vi "3_AdvancedDemo_HHT3.vi"() -> ()   [LabVIEW 2010]
uses:
  Types/HH_UIThread_Data.ctl
  Types/HH_InputChannel.ctl
  _lib/PQ/HydraHarp/HH_RefSource.ctl
  _lib/PQ/HydraHarp/HH_MeasMode.ctl
  _lib/PQ/HydraHarp/hhlib_x86_x64_UIThread.llb/HH_DllPath_global.vi
  <vilib>/Utility/error.llb/DialogType.ctl
  Types/HH_DataProcThread_QCmds.ctl
  Types/HH_DataProcThread_QData.ctl
  Types/HH_VisThread_QCmds.ctl
  Types/HH_VisThread_QData.ctl
  Types/HH_VisThread_Data.ctl
  _lib/PQ/HydraHarp/HH_LibVersion_global.vi
  _lib/PQ/HydraHarp/HH_InitInfo.ctl
  Types/HH_UIThread_Cmds.ctl
panel:
  in  "Settings":bool=TRUE
  in  "Run continuously":bool caption="Conti."
  in  "Start":bool
  in  "Scale":bool
  out "CountRates":i32[](graph)
  in  "HistoAcqTime":dbl=1.0 caption="Int.Time    s" min=0.1 max=360000.0 step=0.1
  in  "AcqTime":i32=360000000 caption="T3Acq.   ms" min=1 max=360000 step=1
  in  "Binning":i32(ring) caption="Resol.      ps" items=["1", "2", "4", "8", "16", "32", "64", "128", "256", "512", "1024", "2048", "4096", "8192", "16384", "32768", "65536", "131072", "262144", "524288", "1048576", "2097152", "4194304", "8388608", "16777216", "33554432"]
  in  "HistoOffset":i32 caption="Offset      ns" min=0 max=500000 step=1
  out "DeltaT":dbl=inf caption="Resol.     ms" format="%.2f"
  in  "BitShift":i32=15 min=0 max=32 step=1
  in  "OvlLevel":i32=65536 caption="Ovl.Level" min=1024 max=65536 step=1024
  in  "StopOvl.":bool=TRUE
  out "TTraceGraph":T1(graph)
  out "HistoGraph":cluster{dbl, "Resol":dbl, "Histos":u32[][]}(graph)
  in  "SyncZeroX":i32=10 caption="ZeroCr.  mV" min=0 max=40 step=1
  in  "SyncDivider":i32(ring)=3 caption="Divider" items=["1", "2", "4", "8", "16"]
  in  "SyncOffset":i32 caption="Offset      ps" min=-99999 max=99999 step=1
  in  "SyncLevel":i32=50 caption="Level      mV" min=0 max=1000 step=1
  in  "Channels":T2[](array[typedef])=[{"Name"="Inp.Chan 1", "Enable"=TRUE, "Offset"=0, "CFDLevel"=50, "ZeroX"=10}, {"Name"="Inp.Chan 2", "Enable"=TRUE, "Offset"=0, "CFDLevel"=50, "ZeroX"=10}, {"Name"="Inp.Chan 3", "Enable"=TRUE, "Offset"=0, "CFDLevel"=50, "ZeroX"=10}, {"Name"="Inp.Chan 4", "Enable"=TRUE, "Offset"=0, "CFDLevel"=50, "ZeroX"=10}, {"Name"="Inp.Chan 5", "Enable"=TRUE, "Offset"=0, "CFDLevel"=50, "ZeroX"=10}, {"Name"="Inp.Chan 6", "Enable"=TRUE, "Offset"=0, "CFDLevel"=50, "ZeroX"=10}, {"Name"="Inp.Chan 7", "Enable"=TRUE, "Offset"=0, "CFDLevel"=50, "ZeroX"=10}, {"Name"="Inp.Chan 8", "Enable"=TRUE, "Offset"=0, "CFDLevel"=50, "ZeroX"=10}] {"ZeroX" min=0 max=40 step=1; "Offset" min=-99999 max=99999 step=1; "CFDLevel" min=0 max=1000 step=1}
  out "SyncRate":string="Sync Rate: 0 cps\n"
  out "OverRun":bool caption="Overrun:"
  out "Status":string="Elements in Q: 0"
  # "Histogram"
  # "Time Trace"
  # "Sync"
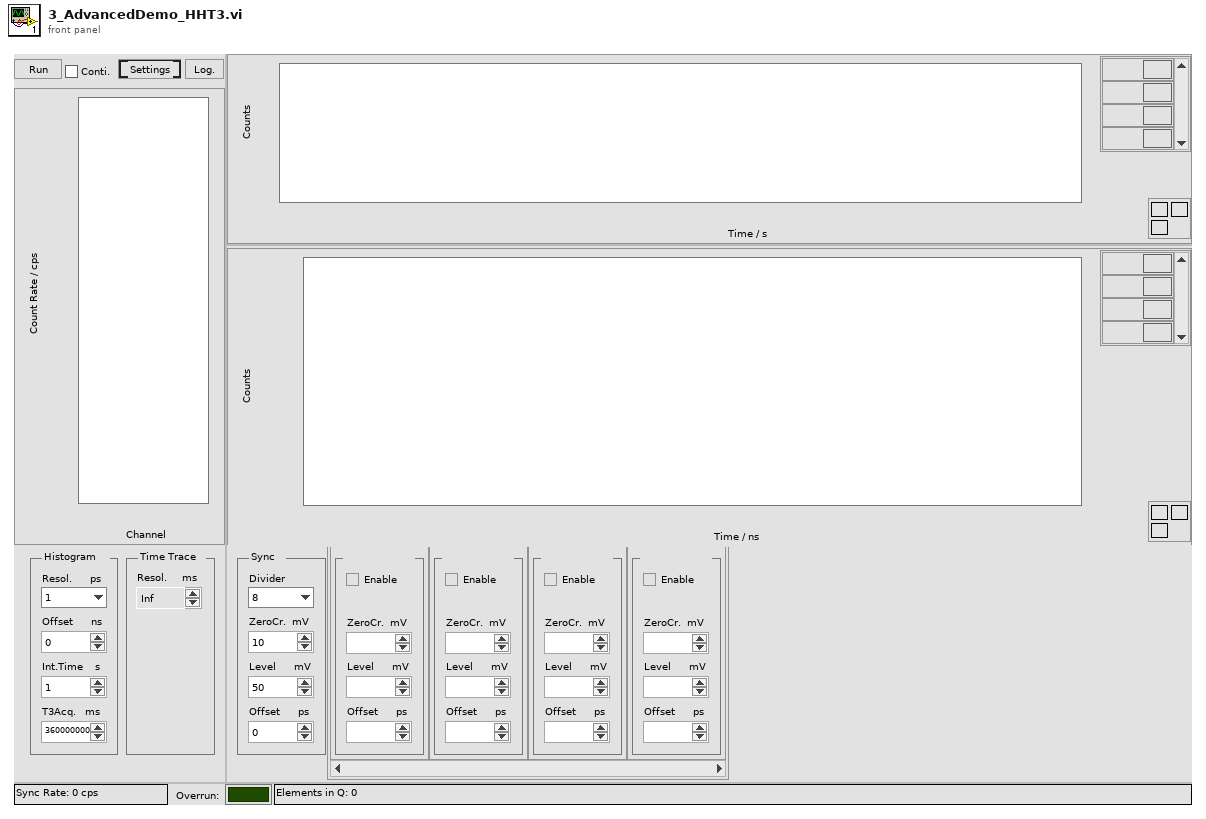
[diagram p1: front panel]
types:
  T1 = cluster{dbl, "Resolution":dbl, "Histogram":u32[][]}
  T2 = typedef "HH_InputChannel.ctl" = cluster{"Name":string, "Enable":bool, "Offset":i32, "CFDLevel":i32, "ZeroX":i32}
  T3 = typedef "HH_DataProcThread_QCmds.ctl" = enum16{"Exit", "Proc", "Init", "SetShift", "SetNumChannels", "SetHistAcqTime"}
  T4 = typedef "HH_VisThread_Data.ctl" = cluster{"Resol":dbl, "DeltaT":dbl, "NumChannels":i32}
  T5 = typedef "HH_VisThread_QData.ctl" = cluster{"Histos":u32[][], "Cmd":T6, "TimeTrace":u32[][], "Bin":i32, "Total bin":u64, "Status":string, "Resol":dbl, "DeltaT":dbl, "nChannels":i32}
  T6 = typedef "HH_VisThread_QCmds.ctl" = enum16{"_none_", "Resol", "nChannels", "DeltaT", "Histo", "TTrace", "Status"}
  T7 = typedef "HH_DataProcThread_QData.ctl" = cluster{"Cmd":T3, "nActual":i32, "Buffer":u32[], "TickCount":u32, "Param":i32}
  T8 = typedef "HH_UIThread_Data.ctl" = cluster{"Init Info":T9, "DevIdx":i32, "SyncDivider":i32, "SyncOffset":i32, "SyncLevel":i32, "Channels":T2[], "CurrentChannels":i32[], "AcqTime":i32, "Binning":i32, "HistoOffset":i32, "HistoLen":i32, "StopOvl.":bool, "OvlLevel":u32, "StartMeas":bool, "HistoLength":i32, "Resolution":dbl, "Run cont.":bool, "Status":string, "SyncRate":i32, "BitShift":i32, "HistoAcqTime":dbl, "SyncZeroX":i32, "SyncRateStart":i32}
  T9 = typedef "HH_InitInfo.ctl" = cluster{"Library Version":string, "Serial No.":string, "Model":string, "Partnum":string, "Version":string, "features":i32, "nchannels":i32, "nummod":i32, "Model Codes":i32[], "Version Codes":i32[], "Base Resolution":dbl, "Bin Steps":i32}
  T10 = typedef "HH_UIThread_Cmds.ctl" = enum16{"Idle", "Init", "SetInpChanEnable", "SetInpChanOffset", "SetInpChanTrg", "SetSyncDivider", "SetSyncTrg", "SetSyncOffset", "SetBinning", "SetHistoOffset", "SetHistoLen", "SetStopOvl", "SetBitShift", "SetHistoAcqTime", "GetRates", "StartMeas", "StopMeas", "AbortMeas", "GetResolution", "GetHisto", "ReadFiFo", "WriteStatus", "Resize", "EnableControls", "DisableControls", "Error", "Exit"}
  T11 = enum8{"Enabled", "Disabled", "Disabled and Grayed Out"}
  T12 = typedef "HH_MeasMode.ctl" = i32
  T13 = typedef "HH_RefSource.ctl" = enum16{"internal", "external"}
  T14 = typedef "DialogType.ctl" = u16
  T15 = cluster{"T0":dbl, "dt":dbl, "TimeTrace_out":u32[][]}
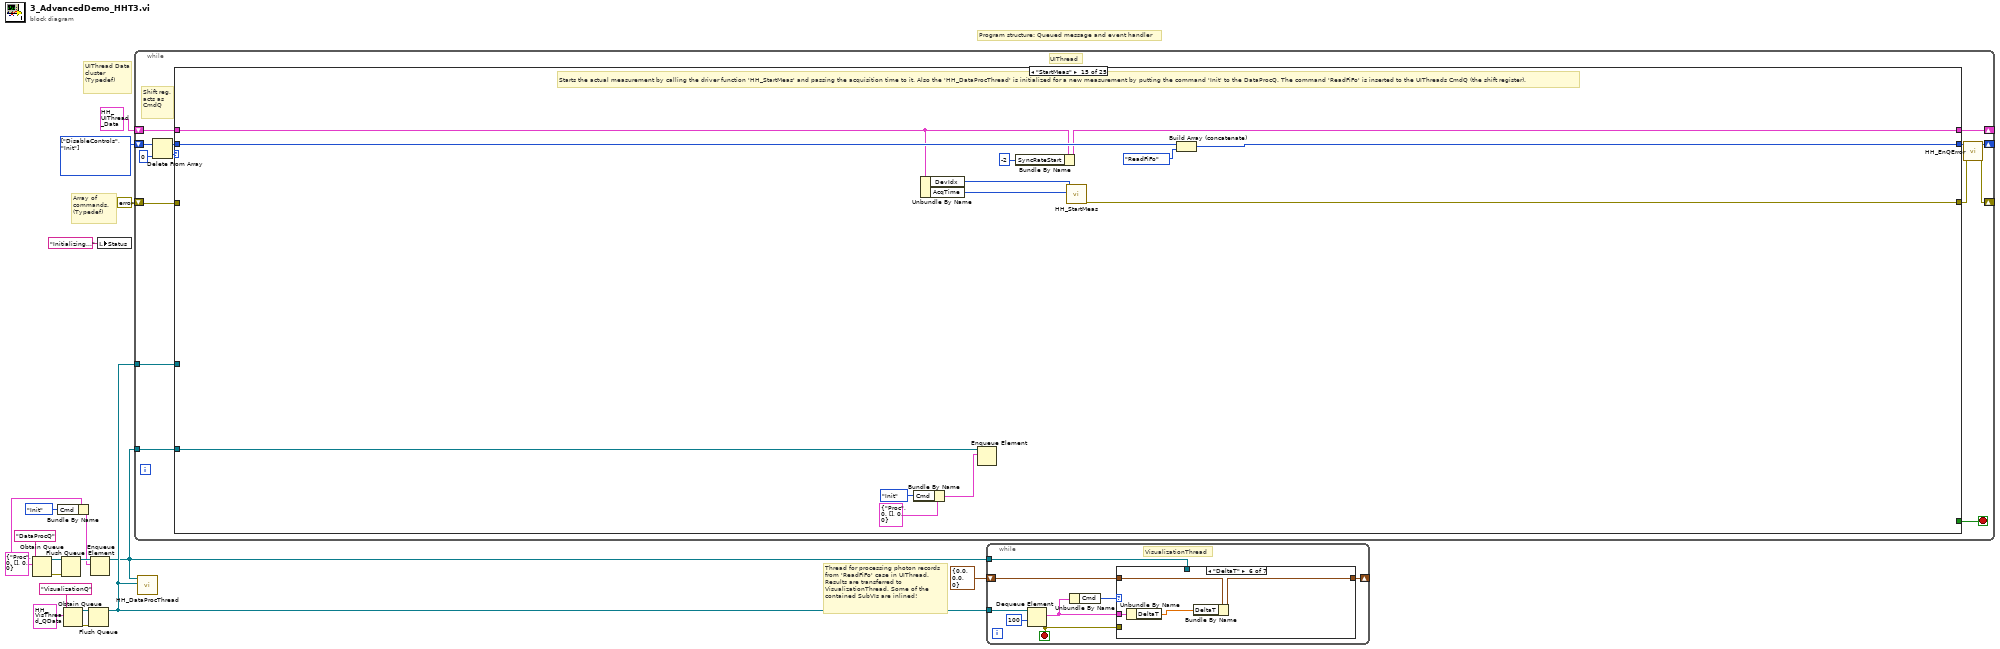
[diagram p0: block diagram]
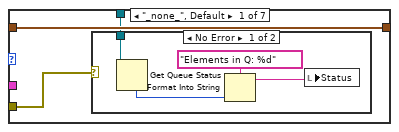
[diagram p2: hidden frame]
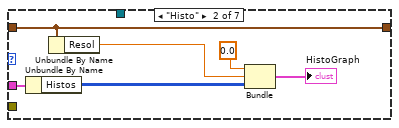
[diagram p4: hidden frame]
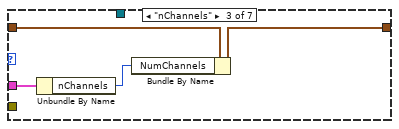
[diagram p5: hidden frame]
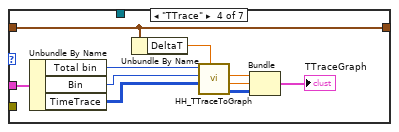
[diagram p6: hidden frame]
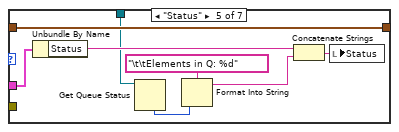
[diagram p7: hidden frame]
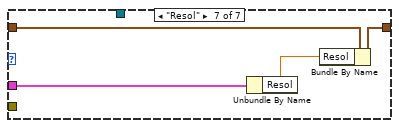
[diagram p8: hidden frame]
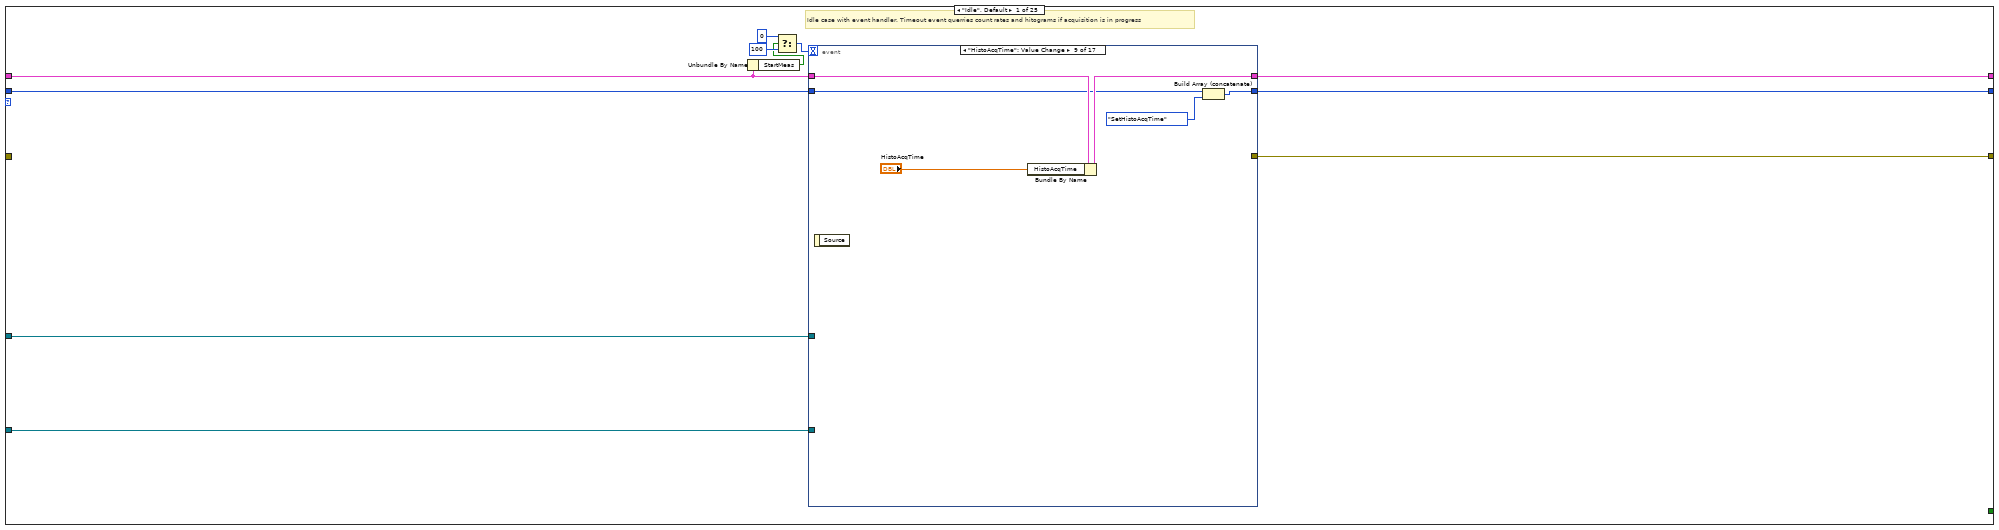
[diagram p9: hidden frame]
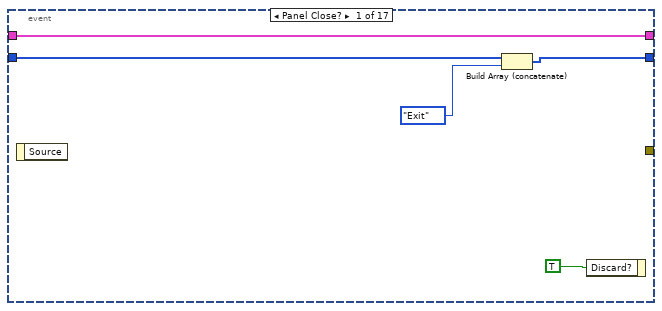
[diagram p10: hidden frame]
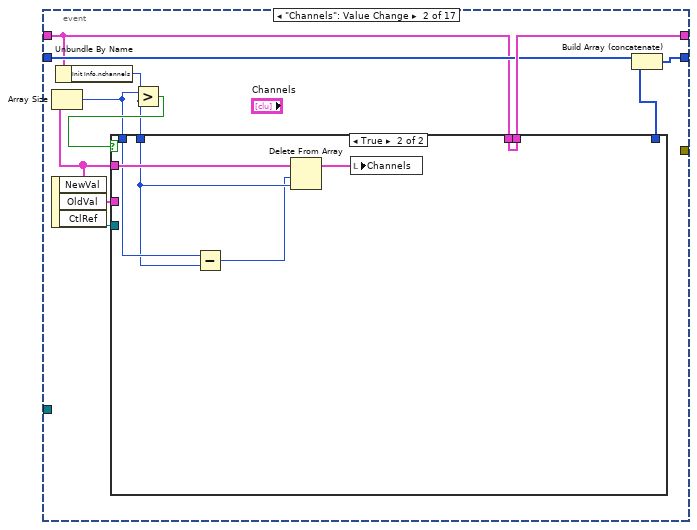
[diagram p11: hidden frame]
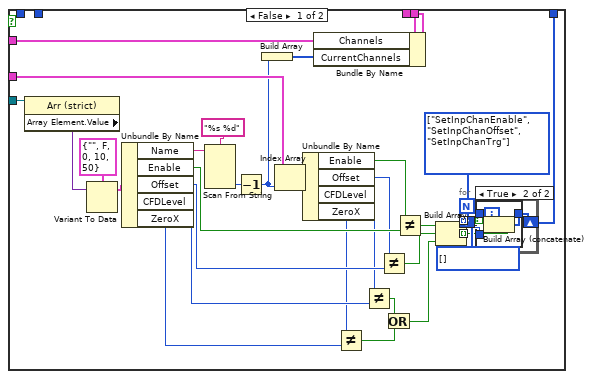
[diagram p12: hidden frame]
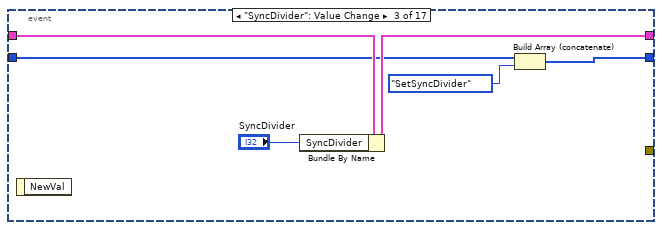
[diagram p14: hidden frame]
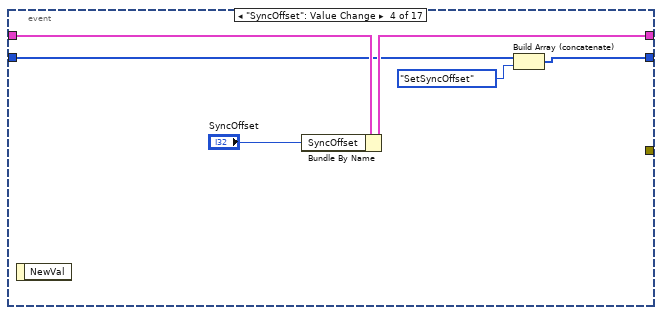
[diagram p15: hidden frame]
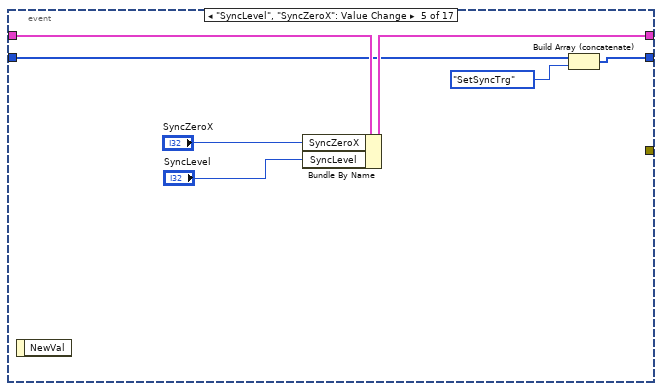
[diagram p16: hidden frame]
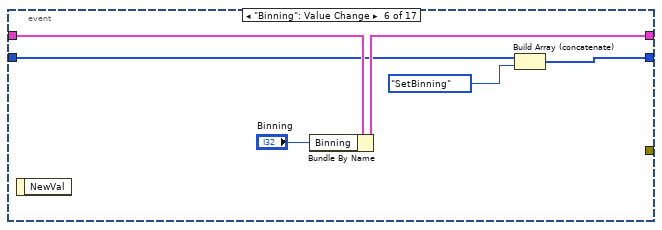
[diagram p17: hidden frame]
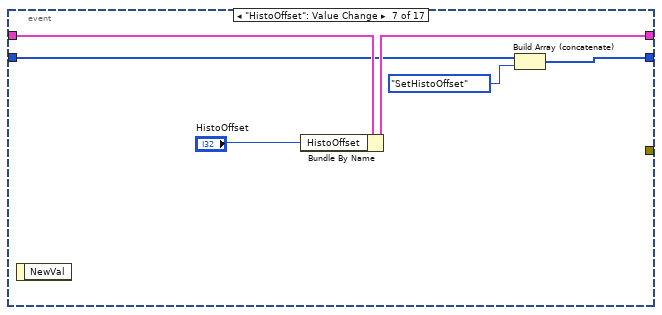
[diagram p18: hidden frame]
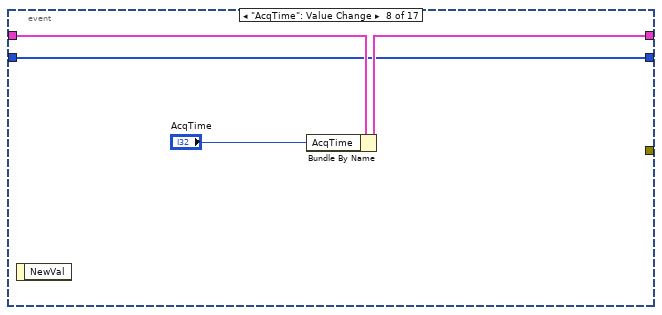
[diagram p19: hidden frame]
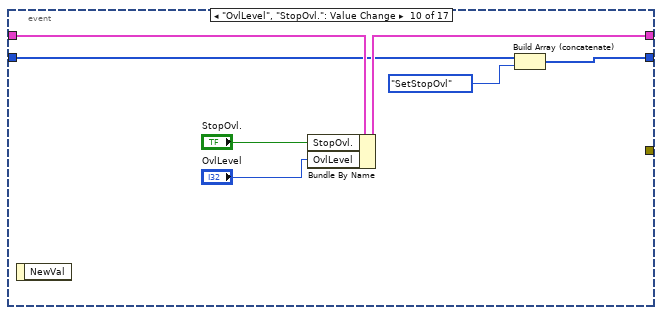
[diagram p20: hidden frame]
diagram:
  w4 = T7 {"Cmd"=enum."Proc", "nActual"=0, "Buffer"=[], "TickCount"=0, "Param"=0} ("MH_DataProcThread_QData")
  w17 = T10[] [enum."DisableControls", enum."Init"] items=["Idle", "Init", "SetInpChanEnable", "SetInpChanOffset", "SetInpChanTrg", "SetSyncDivider", "SetSyncTrg", "SetSyncOffset", "SetBinning", "SetHistoOffset", "SetHistoLen", "SetStopOvl", "SetBitShift", "SetHistoAcqTime", "GetRates", "StartMeas", "StopMeas", "AbortMeas", "GetResolution", "GetHisto", "ReadFiFo", "WriteStatus", "Resize", "EnableControls", "DisableControls", "Error", "Exit"]
  # "Thread for processing photon records from 'ReadFiFo' case in UIThread. Results are transferred to VisualizationThread. Some of the contained SubVIs are inlined!"
  # "Array of commands.\n(Typedef)"
  # "Program structure: Queued message and event handler"
  # "UIThread Data cluster\n(Typedef)"
  n1 = Obtain Queue(name (unnamed)="DataProcQ", element data type=w4) -> (queue out=w14:refnum<queue>, error out=w13:errorcluster)  [unwired: 3 in, 1 out]
  n2 = Bundle By Name(cluster=w4, "Cmd"=HH_DataProcThread_QCmds."Init") -> (w2:T7)
  n3 = Flush Queue(queue=w14, error in (no error)=w13) -> (queue out=w5:refnum<queue>)  [unwired: 2 out]
  n4 = Obtain Queue(name (unnamed)="VisualizationQ", element data type=T5 {"Histos"=[], "Cmd"=enum."_none_", "TimeTrace"=[], "Bin"=0, "Total bin"=0, "Status"="", "Resol"=0.0, "DeltaT"=0.0, "nChannels"=0} ("MH_GUIThread_QData")) -> (queue out=w12:refnum<queue>, error out=w11:errorcluster)  [unwired: 3 in, 1 out]
  n5 = Flush Queue(queue=w12, error in (no error)=w11) -> (queue out=w7:refnum<queue>)  [unwired: 2 out]
  n6 = Enqueue Element(queue=w5, element=w2) -> (queue out=w1:refnum<queue>)  [unwired: 2 in, 2 out]
  n7 = local write "Status"("Initializing..." ("Status")) -> ()
  n8 = while {
    shift-right: [w21] -> _
    shift-left: w17 -> [w28]
    shift-right: [w31] -> _
    shift-left: T8 {"Init Info"={"Library Version"="", "Serial No."="", "Model"="", "Partnum"="", "Version"="", "features"=0, "nchannels"=0, "nummod"=0, "Model Codes"=[], "Version Codes"=[], "Base Resolution"=0.0, "Bin Steps"=0}, "DevIdx"=0, "SyncDivider"=1, "SyncOffset"=0, "SyncLevel"=50, "Channels"=[], "CurrentChannels"=[], "AcqTime"=1, "Binning"=1, "HistoOffset"=1, "HistoLen"=1024, "StopOvl."=FALSE, "OvlLevel"=1024, "StartMeas"=FALSE, "HistoLength"=0, "Resolution"=0.0, "Run cont."=FALSE, "Status"="", "SyncRate"=0, "BitShift"=0, "HistoAcqTime"=0.0, "SyncZeroX"=10, "SyncRateStart"=0} -> [w30]
    shift-right: [w23] -> _
    shift-left: errorcluster {"status"=FALSE, "code"=0, "source"=""} ("error IO") -> [w29]
    tunnel: w1 -> [w20]
    tunnel: w7 -> [w19]
    stop <- w32 stop-if-true
    # "Shift reg.\nacts as\nCmdQ"
    # "UIThread"
    n9 = Delete From Array(array=w28, index=0) -> (deleted portion=w26:T10, array with subset deleted=w25:T10[])  [unwired: 1 in]
    n10 = case shown="\"StartMeas\"" w26 {
      tunnel: [w43 w283 w307 w321 w335 w352 w361 w363 w370 w378 w385 w405 w417 w426 w504 w509 w522 w539 w540 w566 w579 w586 w598 w604 w610] -> w22
      tunnel: [_ _ _ _ _ _ _ _ _ _ _ _ _ _ _ _ _ _ _ _ _ _ _ _ TRUE] -> w32
      tunnel: [w42 w264 w310 w324 w338 w354 w362 w367 w374 w379 w386 w390 w407 w429 w496 w512 w524 w535 w550 w565 w567 w585 w597 w605 w613] -> w31
      tunnel: w30 -> [w39 w269 w310 w324 w338 w354 w362 w367 w374 w379 w386 w390 w407 w425 w497 w513 w525 w536 w550 w565 w567 w585 w597 w605 w613]
      tunnel: [w40 w288 w308 w322 w336 w350 w360 w366 w373 w377 w384 _ _ w435 w507 w515 w527 w537 w545 _ _ _ _ _ w611] -> w24
      tunnel: w29 -> [_ _ _ _ _ _ _ _ _ _ _ _ _ _ _ _ _ _ _ _ _ _ _ w606 _]
      tunnel: w25 -> [w41 w285 w307 w321 w335 w352 w361 w363 w369 w378 w385 w405 w417 w427 w505 w510 w522 w539 w541 w566 w579 w586 w598 _ w610]
      tunnel: w20 -> [w34 w262 _ _ _ _ _ _ _ _ _ w391 w408 _ w501 _ _ _ w542 _ _ _ _ _ w609]
      tunnel: w19 -> [w33 w254 _ _ _ _ _ _ _ _ _ w392 _ _ _ _ _ w532 _ _ _ _ _ _ w608]
      frame "Idle", Default {
        # "Idle case with event handler. Timeout event querries count rates and hitograms if acquisition is in progress"
        n11 = Unbundle By Name(w39) -> ("StartMeas"=w37:bool)
        n12 = Select(t=0, s=w37, f=100) -> (s? t:f=w36:i32)
        n13 = event shown="[8] \"HistoAcqTime\": Value Change" {
          selector: _ -> [_ _ _ _ _ _ _ _ _ _ _ _ _ _ _ _ _]
          dyn-events: _ -> [_ _ _ _ _ _ _ _ _ _ _ _ _ _ _ _ _]
          timeout: w36 -> [_ _ _ _ _ _ _ _ _ _ _ _ _ _ _ _ _]
          tunnel: [w44 w54 w105 w111 w118 w125 w131 w136 w141 w148 w163 w181 w193 w211 w217 w225 w235] -> w43
          tunnel: [w47 w57 w109 w115 w122 w128 w134 w138 w144 w151 w162 w185 w192 w209 w216 w224 w238] -> w42
          tunnel: w39 -> [w47 w53 w110 w116 w123 w129 w135 w139 w145 w152 w162 w186 w190 w210 w216 w224 w238]
          tunnel: w41 -> [w46 w56 w107 w113 w120 w127 w133 w136 w142 w150 w164 w182 w194 w211 w217 w225 w236]
          tunnel: [_ _ _ _ _ _ _ _ _ _ w158 _ _ _ _ _ _] -> w40
          tunnel: w34 -> [_ _ _ _ _ _ _ _ _ _ _ _ _ _ _ _ _]
          tunnel: w33 -> [_ _ _ _ _ _ _ _ _ _ _ _ _ _ _ _ _]
          event Panel Close? {
            n14 = event-data() -> ()  [unwired: 1 in, 1 out]
            n15 = Build Array (concatenate)(w46, HH_UIThread_Cmds."Exit") -> (w44:T10[])
            n16 = event-data("Discard?"=TRUE) -> ()  [unwired: 1 in, 1 out]
          }
          event "Channels": Value Change {
            n17 = event-data() -> ("NewVal"=w52:T2[], "OldVal"=w58:T2[], "CtlRef"=w59:refnum<vi>)  [unwired: 1 in]
            n18 = Array Size(array=w52) -> (size(s)=w49:i32)
            n19 = Unbundle By Name(w53) -> ("Init Info.nchannels"=w50:i32)
            n20 = Greater?(x=w49, y=w50) -> (0:w51:bool)
            n21 = case shown="True" w51 {
              tunnel: w59 -> [w90 _]
              tunnel: w58 -> [w84 _]
              tunnel: [w67 w104] -> w57
              tunnel: [w65 _] -> w55
              tunnel: w53 -> [w62 w104]
              tunnel: w52 -> [w61 w103]
              tunnel: w50 -> [_ w101]
              tunnel: w49 -> [_ w102]
              frame False {
                w60 = T10[] [] items=["Idle", "Init", "SetInpChanEnable", "SetInpChanOffset", "SetInpChanTrg", "SetSyncDivider", "SetSyncTrg", "SetSyncOffset", "SetBinning", "SetHistoOffset", "SetHistoLen", "SetStopOvl", "SetBitShift", "SetHistoAcqTime", "GetRates", "StartMeas", "StopMeas", "AbortMeas", "GetResolution", "GetHisto", "ReadFiFo", "WriteStatus", "Resize", "EnableControls", "DisableControls", "Error", "Exit"] ("Array")
                w68 = T10[] [enum."SetInpChanEnable", enum."SetInpChanOffset", enum."SetInpChanTrg"] items=["Idle", "Init", "SetInpChanEnable", "SetInpChanOffset", "SetInpChanTrg", "SetSyncDivider", "SetSyncTrg", "SetSyncOffset", "SetBinning", "SetHistoOffset", "SetHistoLen", "SetStopOvl", "SetBitShift", "SetHistoAcqTime", "GetRates", "StartMeas", "StopMeas", "AbortMeas", "GetResolution", "GetHisto", "ReadFiFo", "WriteStatus", "Resize", "EnableControls", "DisableControls", "Error", "Exit"]
                n22 = property class="Arr (strict)"(reference=w90) -> ("Array Element.Value"=w89:variant)  [unwired: 1 in, 2 out]
                n23 = Variant To Data(Variant=w89, type=T2 {"Name"="", "Enable"=FALSE, "Offset"=0, "CFDLevel"=10, "ZeroX"=50} ("Channel")) -> (data=w66:cluster{})  [unwired: 1 in, 1 out]
                n24 = Unbundle By Name(w66) -> ("Name"=w87:string, "Enable"=w81:bool, "Offset"=w79:i32, "CFDLevel"=w77:i32, "ZeroX"=w75:i32)
                n25 = Scan From String(format string="%s %d", input string=w87) -> (output 2=w85:i32)  [unwired: 5 in, 3 out]
                n26 = Decrement(x=w85) -> (x-1=w64:i32)
                n27 = Build Array(w64) -> (w63:i32[])
                n28 = Index Array(array=w84, index=w64) -> (element=w83:T2)
                n29 = Unbundle By Name(w83) -> ("Enable"=w82:bool, "Offset"=w80:i32, "CFDLevel"=w78:i32, "ZeroX"=w76:i32)
                n30 = Bundle By Name(cluster=w62, "Channels"=w61, "CurrentChannels"=w63) -> (w67:T8)
                n31 = Not Equal?(x=w76, y=w75) -> (x != y?=w70:bool)
                n32 = Not Equal?(x=w78, y=w77) -> (x != y?=w71:bool)
                n33 = Not Equal?(x=w80, y=w79) -> (x != y?=w73:bool)
                n34 = Or(x=w71, y=w70) -> (x .or. y?=w69:bool)
                n35 = Not Equal?(x=w82, y=w81) -> (x != y?=w74:bool)
                n36 = Build Array(w74, w73, w69) -> (w72:bool[])
                n37 = for {
                  tunnel: w72 -> [w93] mode=indexing
                  tunnel: w68 -> [w94] mode=indexing
                  shift-right: [w91] -> w65
                  shift-left: w60 -> [w92]
                  n38 = case shown="True" w93 {
                    tunnel: w92 -> [w95 w97]
                    tunnel: w94 -> [_ w96]
                    tunnel: [w95 w98] -> w91
                    frame False {
                    }
                    frame True {
                      n39 = Build Array (concatenate)(w97, w96) -> (w98:T10[])
                    }
                  }
                }
              }
              frame True {
                n40 = Subtract(x=w102, y=w101) -> (x-y=w100:i32)
                n41 = Delete From Array(array=w103, length=w100, index=w101) -> (array with subset deleted=w99:T2[])  [unwired: 1 out]
                n42 = local write "Channels"(w99) -> ()
              }
            }
            n43 = Build Array (concatenate)(w56, w55) -> (w54:T10[])
          }
          event "SyncDivider": Value Change {
            n44 = event-data() -> ()  [unwired: 1 in, 1 out]
            n45 = Bundle By Name(cluster=w110, "SyncDivider"="SyncDivider") -> (w109:T8)
            n46 = Build Array (concatenate)(w107, HH_UIThread_Cmds."SetSyncDivider") -> (w105:T10[])
          }
          event "SyncOffset": Value Change {
            n47 = event-data() -> ()  [unwired: 1 in, 1 out]
            n48 = Bundle By Name(cluster=w116, "SyncOffset"="SyncOffset") -> (w115:T8)
            n49 = Build Array (concatenate)(w113, HH_UIThread_Cmds."SetSyncOffset") -> (w111:T10[])
          }
          event "SyncLevel", "SyncZeroX": Value Change {
            n50 = event-data() -> ()  [unwired: 1 in, 1 out]
            n51 = Bundle By Name(cluster=w123, "SyncZeroX"="SyncZeroX", "SyncLevel"="SyncLevel") -> (w122:T8)
            n52 = Build Array (concatenate)(w120, HH_UIThread_Cmds."SetSyncTrg") -> (w118:T10[])
          }
          event "Binning": Value Change {
            n53 = event-data() -> ()  [unwired: 1 in, 1 out]
            n54 = Bundle By Name(cluster=w129, "Binning"="Binning") -> (w128:T8)
            n55 = Build Array (concatenate)(w127, HH_UIThread_Cmds."SetBinning") -> (w125:T10[])
          }
          event "HistoOffset": Value Change {
            n56 = event-data() -> ()  [unwired: 1 in, 1 out]
            n57 = Bundle By Name(cluster=w135, "HistoOffset"="HistoOffset") -> (w134:T8)
            n58 = Build Array (concatenate)(w133, HH_UIThread_Cmds."SetHistoOffset") -> (w131:T10[])
          }
          event "AcqTime": Value Change {
            n59 = event-data() -> ()  [unwired: 1 in, 1 out]
            n60 = Bundle By Name(cluster=w139, "AcqTime"="AcqTime") -> (w138:T8)
          }
          event "HistoAcqTime": Value Change {
            n61 = event-data() -> ()  [unwired: 1 in, 1 out]
            n62 = Bundle By Name(cluster=w145, "HistoAcqTime"="HistoAcqTime") -> (w144:T8)
            n63 = Build Array (concatenate)(w142, HH_UIThread_Cmds."SetHistoAcqTime") -> (w141:T10[])
          }
          event "OvlLevel", "StopOvl.": Value Change {
            n64 = event-data() -> ()  [unwired: 1 in, 1 out]
            n65 = Bundle By Name(cluster=w152, "StopOvl."="StopOvl.", "OvlLevel"="OvlLevel") -> (w151:T8)
            n66 = Build Array (concatenate)(w150, HH_UIThread_Cmds."SetStopOvl") -> (w148:T10[])
          }
          event Timeout {
            n67 = event-data() -> ()  [unwired: 1 in, 1 out]
            n68 = Unbundle By Name(w162) -> ("DevIdx"=w160:i32, "StartMeas"=w161:bool, "BitShift"=w157:i32, "SyncRate"=w156:i32)
            n69 = case shown="True" w161 {
              tunnel: w160 -> [_ w180]
              tunnel: [_ w178] -> w159
              tunnel: [_ w175] -> w158
              frame False {
              }
              frame True {
                w176 = T10[] [enum."ReadFiFo"] items=["Idle", "Init", "SetInpChanEnable", "SetInpChanOffset", "SetInpChanTrg", "SetSyncDivider", "SetSyncTrg", "SetSyncOffset", "SetBinning", "SetHistoOffset", "SetHistoLen", "SetStopOvl", "SetBitShift", "SetHistoAcqTime", "GetRates", "StartMeas", "StopMeas", "AbortMeas", "GetResolution", "GetHisto", "ReadFiFo", "WriteStatus", "Resize", "EnableControls", "DisableControls", "Error", "Exit"]
                w177 = T10[] [enum."StopMeas"] items=["Idle", "Init", "SetInpChanEnable", "SetInpChanOffset", "SetInpChanTrg", "SetSyncDivider", "SetSyncTrg", "SetSyncOffset", "SetBinning", "SetHistoOffset", "SetHistoLen", "SetStopOvl", "SetBitShift", "SetHistoAcqTime", "GetRates", "StartMeas", "StopMeas", "AbortMeas", "GetResolution", "GetHisto", "ReadFiFo", "WriteStatus", "Resize", "EnableControls", "DisableControls", "Error", "Exit"]
                n70 = call "HH_CTCStatus.vi"("devidx"=w180) -> ("error out"=w175:errorcluster, "ctcstatus"=w179:i32)  [unwired: 8 in, 1 out]
                n71 = Not Equal To 0?(x=w179) -> (x != 0?=w174:bool)
                n72 = Select(t=w177, s=w174, f=w176) -> (s? t:f=w178:T10[])
              }
            }
            n73 = call "CalcRate.vi"("Refresh(ms)"=u32 100) -> ("updated?"=w154:bool)  [unwired: 8 in, 2 out]
            n74 = case shown="True" w154 {
              tunnel: w157 -> [_ w167]
              tunnel: w156 -> [_ w166]
              tunnel: [_ HH_UIThread_Cmds."GetRates"] -> w155
              frame False {
              }
              frame True {
                n75 = To Double Precision Float(number=w166) -> (double precision float=w171:dbl)
                n76 = To Double Precision Float(number=w167) -> (double precision float=w172:dbl)
                n77 = Power Of 2(x=w172) -> (2^x=w170:dbl)
                n78 = Multiply(x=w170, y=1000.0) -> (x*y=w169:dbl)
                n79 = Divide(x=w169, y=w171) -> (x/y=w173:dbl)
                n80 = local write "DeltaT"(w173) -> ()
              }
            }
            n81 = Build Array (concatenate)(w164, w159, w155) -> (w163:T10[])
          }
          event "BitShift": Value Change {
            n82 = event-data() -> ()  [unwired: 1 in, 1 out]
            n83 = Bundle By Name(cluster=w186, "BitShift"="BitShift") -> (w185:T8)
            n84 = Build Array (concatenate)(w182, HH_UIThread_Cmds."SetBitShift") -> (w181:T10[])
          }
          event "Start": Value Change {
            n85 = event-data() -> ()  [unwired: 1 in, 1 out]
            n86 = Unbundle By Name(w190) -> ("SyncRate"=w189:i32)
            n87 = Greater Or Equal?(x=w189, y=10) -> (x >= y?=w187:bool)
            n88 = case shown="True" w187 {
              selector: w187 -> [w196 _]
              tunnel: w194 -> [w198 w207]
              tunnel: [w198 w205] -> w193
              tunnel: [w197 w204] -> w192
              tunnel: "Start" -> [_ w203]
              tunnel: w190 -> [w197 w199]
              frame False {
                n89 = local write "Start"(w196) -> ()
                n90 = One Button Dialog(message="SyncRate too low!!!" ("Status")) -> ()  [unwired: 1 in, 1 out]
              }
              frame True {
                w202 = T10[] [enum."SetBitShift", enum."SetHistoAcqTime", enum."StartMeas"] items=["Idle", "Init", "SetInpChanEnable", "SetInpChanOffset", "SetInpChanTrg", "SetSyncDivider", "SetSyncTrg", "SetSyncOffset", "SetBinning", "SetHistoOffset", "SetHistoLen", "SetStopOvl", "SetBitShift", "SetHistoAcqTime", "GetRates", "StartMeas", "StopMeas", "AbortMeas", "GetResolution", "GetHisto", "ReadFiFo", "WriteStatus", "Resize", "EnableControls", "DisableControls", "Error", "Exit"]
                # "When starting a measurement three commands are added to the CmdQ (the shift register) and get processed in the corresponding cases of the UIThread: \n\n1. 'SetBitShift': Parameter determining the  temporal resolution of the photons time trace\n\n2. 'SetHistoAcqTime': The time interval for accumulating a histogram from the photon stream (for details refer to the corresponding case)\n\n3. 'StartMeas': Starts the actual measurement (for details refer to the corresponding case)"
                n91 = Bundle By Name(cluster=w199, "StartMeas"=w203) -> (w204:T8)
                n92 = Build Array(HH_UIThread_Cmds."AbortMeas") -> (w200:T10[])
                n93 = Select(t=w202, s=w203, f=w200) -> (s? t:f=w206:T10[])
                n94 = Build Array (concatenate)(w207, w206) -> (w205:T10[])
              }
            }
          }
          event "Run continuously": Value Change {
            n95 = event-data() -> ()  [unwired: 1 in, 1 out]
            n96 = Bundle By Name(cluster=w210, "Run cont."="Run continuously") -> (w209:T8)
          }
          event "Scale": Value Change {
            n97 = event-data() -> ()  [unwired: 1 in, 1 out]
            n98 = Select(t=u8 0 ("Y Scale.Mapping Mode"), s="Scale", f=u8 1 ("Y Scale.Mapping Mode")) -> (s? t:f=w212:u8)
            n99 = property on="HistoGraph" class="WFGraph (strict)"("YScale.Mapping Mode"=w212) -> ()  [unwired: 2 in, 2 out]
          }
          event "Settings": Value Change {
            n100 = event-data() -> ()  [unwired: 1 in, 1 out]
            n101 = property on="Splitter" class="Splitter"() -> ("Position"=w223:i32)  [unwired: 2 in, 2 out]
            n102 = Select(t=237 ("PosT"), s="Settings", f=0 ("PosF")) -> (s? t:f=w220:i32)
            n103 = Subtract(x=w223, y=w220) -> (x-y=w219:i32)
            n104 = while {
              shift-right: [w234] -> _
              shift-left: w219 -> [w227]
              i -> [w233]
              stop <- w230 stop-if-true
              n105 = property on="Splitter 4" class="Splitter"("Position"=w227) -> (error out=w226:errorcluster)  [unwired: 2 in, 1 out]
              n106 = Greater Or Equal?(x=w233, y=10) -> (x >= y?=w231:bool)
              n107 = Decrement(x=w227) -> (x-1=w234:i32)
              n108 = Unbundle(w226) -> ("status"=w229:bool)  [unwired: 2 out]
              n109 = Not(x=w229) -> (.not. x?=w228:bool)
              n110 = Or(x=w228, y=w231) -> (x .or. y?=w230:bool)
            }
          }
          event Panel Resize {
            n111 = event-data() -> ()  [unwired: 1 in, 1 out]
            n112 = Build Array (concatenate)(w236, HH_UIThread_Cmds."Resize") -> (w235:T10[])
          }
        }
      }
      frame "Init" {
        w245 = T12 3 items=["Histo"=0, "T2"=2, "T3"=3, "Conti"=8]  # mode
        w244 = HH_RefSource."internal"  # refsource
        w252 = 1.0 ("HistoAcqTime")
        w253 = 15 ("Value (Signaling)")
        w271 = FALSE ("Run cont.")
        w273 = FALSE ("StartMeas")
        w274 = 65536 ("OvlLevel")
        w275 = TRUE ("StopOvl.")
        w276 = 360000000 ("AcqTime")
        w277 = 0 ("HistoOffset")
        w278 = 0 ("Binning")
        w279 = 50 ("SyncLevel")
        w280 = 10 ("SyncZeroX")
        w281 = 0 ("SyncOffset")
        w282 = 3 ("SyncDivider")
        w284 = T10[] [enum."SetSyncDivider", enum."SetSyncOffset", enum."SetSyncTrg", enum."SetInpChanEnable", enum."SetInpChanOffset", enum."SetInpChanTrg", enum."SetBinning", enum."SetHistoOffset", enum."Resize", enum."EnableControls", enum."GetRates", enum."SetBitShift", enum."SetHistoAcqTime", enum."WriteStatus"] items=["Idle", "Init", "SetInpChanEnable", "SetInpChanOffset", "SetInpChanTrg", "SetSyncDivider", "SetSyncTrg", "SetSyncOffset", "SetBinning", "SetHistoOffset", "SetHistoLen", "SetStopOvl", "SetBitShift", "SetHistoAcqTime", "GetRates", "StartMeas", "StopMeas", "AbortMeas", "GetResolution", "GetHisto", "ReadFiFo", "WriteStatus", "Resize", "EnableControls", "DisableControls", "Error", "Exit"]
        # "100 x 60 x 60 x 1000 = 100 h"
        # "Init all FP controls and corresponding copy in UIThread Data cluster"
        # "EnQ list of commands"
        # "Array with Inp.Chan."
        # "Initialization: 1. Init HW -> get # of channels -> make array for Inp.Channels\n2. Init all FP controls and corresponding fields in UIThread Data cluster\n3. EnQ list of commands for further initialization"
        n113 = call <vilib>:"Error Cluster From Error Code.vi"("is warning? (False)"=FALSE, "show call chain? (False)"=TRUE, "error message (\"\")"="DLL not found!" ("error message (\"\")"), "error code (0)"=5000) -> ("error out"=w246:errorcluster)  [unwired: 5 in]
        n114 = call "GetDLLPath.vi"("DllName_32bit"="HHLib.dll" ("name or relative path"), "DllName_64bit"="HHLib64.dll" ("name or relative path")) -> ("file exists?"=w248:bool, "DLLPath"=w249:path)  [unwired: 8 in]
        n115 = global write "HH_DllPath_global.vi" "DllPath"(w249) -> ()
        n116 = Select(t=errorcluster {"status"=FALSE, "code"=0, "source"=""} ("error IO"), s=w248, f=w246) -> (s? t:f=w265:errorcluster)
        n117 = global read "HH_LibVersion_global.vi" "Library Version"() -> (w243:string)
        n118 = Build Array (concatenate)(w285, w284) -> (w283:T10[])
        n119 = call "InitHH_UIThread.vi"("error in (no error)"=w265, "mode"=w245, "refsource"=w244, "Library Version"=w243) -> ("error out"=w288:errorcluster, "Init Info"=w291:T9, "DevIdx"=w290:i32)  [unwired: 5 in]
        n120 = local write "SyncDivider"(w282) -> ()
        n121 = local write "SyncOffset"(w281) -> ()
        n122 = local write "SyncZeroX"(w280) -> ()
        n123 = local write "SyncLevel"(w279) -> ()
        n124 = local write "Binning"(w278) -> ()
        n125 = local write "HistoOffset"(w277) -> ()
        n126 = Bundle By Name(cluster=w269, "DevIdx"=w290, "Init Info"=w291, "Status"="Initialized!") -> (w268:T8)
        n127 = Unbundle By Name(w268) -> ("Init Info.Bin Steps"=w267:i32, "Init Info.nchannels"=w255:i32)
        n128 = for {
          N: w255 -> [_]
          tunnel: T2 {"Name"="", "Enable"=FALSE, "Offset"=0, "CFDLevel"=10, "ZeroX"=50} ("Channel") -> [w303]
          tunnel: [w302] -> w287 mode=indexing
          tunnel: [w292] -> w286 mode=indexing
          i -> [w292]
          # "Init values for Inp. Channels"
          n129 = Increment(x=w292) -> (x+1=w295:i32)
          n130 = Format Into String(format string="Inp.Chan %d", w295) -> (resulting string=w300:string)  [unwired: 2 in, 1 out]
          n131 = Format Into String(format string="Ch.%d", w295) -> (resulting string=w293:string)  [unwired: 2 in, 1 out]
          n132 = Bundle By Name(cluster=w303, "Name"=w300, "Enable"=TRUE, "Offset"=0, "CFDLevel"=50 ("CFDZeroX"), "ZeroX"=10 ("CFDLevel")) -> (w302:T2)
          n133 = property on="HistoGraph" class="WFGraph (strict)"("Active Plot"=w292, "Plot.Plot Name"=w293) -> ()  [unwired: 2 in, 2 out]
          n134 = property on="TTraceGraph" class="WFGraph (strict)"("Active Plot"=w292, "Plot.Plot Name"=w293) -> ()  [unwired: 2 in, 2 out]
        }
        n135 = Bundle By Name(cluster=T5 {"Histos"=[], "Cmd"=enum."_none_", "TimeTrace"=[], "Bin"=0, "Total bin"=0, "Status"="", "Resol"=0.0, "DeltaT"=0.0, "nChannels"=0} ("MH_GUIThread_QData"), "Cmd"=HH_VisThread_QCmds."nChannels", "nChannels"=w255) -> (w257:T5)
        n136 = call "HH_CalcBinningValues.vi"("Bin Steps"=w267) -> ("BinningValues"=w272:cluster{"String":string, "Value":i32}[])  [unwired: 10 in]
        n137 = property on="Binning" class="Ring (strict)"("StringsAndValues[]"=w272) -> ()  [unwired: 2 in, 2 out]
        n138 = Bundle By Name(cluster=T7 {"Cmd"=enum."Proc", "nActual"=0, "Buffer"=[], "TickCount"=0, "Param"=0} ("MH_DataProcThread_QData"), "Param"=w255, "Cmd"=HH_DataProcThread_QCmds."SetNumChannels") -> (w261:T7)
        n139 = Enqueue Element(queue=w254, element=w257) -> ()  [unwired: 2 in, 3 out]
        n140 = Enqueue Element(queue=w262, element=w261) -> ()  [unwired: 2 in, 3 out]
        n141 = local write "Channels"(w287) -> ()
        n142 = Bundle By Name(cluster=w268, "Channels"=w287, "CurrentChannels"=w286, "SyncDivider"=w282, "SyncOffset"=w281, "SyncZeroX"=w280, "SyncLevel"=w279, "Binning"=w278, "HistoOffset"=w277, "AcqTime"=w276, "StopOvl."=w275, "OvlLevel"=w274, "StartMeas"=w273, "Run cont."=w271, "BitShift"=w253, "HistoAcqTime"=w252) -> (w264:T8)
        n143 = local write "StopOvl."(w275) -> ()
        n144 = local write "OvlLevel"(w274) -> ()
        n145 = local write "Start"(w273) -> ()
        n146 = local write "Run continuously"(w271) -> ()
        n147 = local write "BitShift"(w253) -> ()
        n148 = local write "AcqTime"(w276) -> ()
        n149 = local write "HistoAcqTime"(w252) -> ()
        n150 = property on="Settings" class="Bool (strict)"("Val(Sgnl)"=TRUE ("Value (Signaling)")) -> ()  [unwired: 2 in, 2 out]
        n151 = property on="Scale" class="Bool (strict)"("Val(Sgnl)"=FALSE ("Value (Signaling)")) -> ()  [unwired: 2 in, 2 out]
      }
      frame "SetInpChanEnable" {
        n152 = Unbundle By Name(w310) -> ("DevIdx"=w309:i32, "Channels"=w304:T2[], "CurrentChannels"=w305:i32[])
        n153 = for {
          tunnel: w309 -> [w317]
          shift-right: [w316] -> w308
          shift-left: errorcluster {"status"=FALSE, "code"=0, "source"=""} ("error out") -> [w315]
          tunnel: w305 -> [w311] mode=indexing
          tunnel: w304 -> [w314]
          n154 = Index Array(array=w314, index=w311) -> (element=w313:T2)
          n155 = Unbundle By Name(w313) -> ("Enable"=w312:bool)
          n156 = call "HH_SetInputChannelEnable.vi"("error in (no error)"=w315, "enable"=w312, "channel"=w311, "devidx"=w317) -> ("error out"=w316:errorcluster)  [unwired: 6 in, 1 out]
        }
      }
      frame "SetInpChanOffset" {
        n157 = Unbundle By Name(w324) -> ("DevIdx"=w323:i32, "Channels"=w318:T2[], "CurrentChannels"=w319:i32[])
        n158 = for {
          tunnel: w323 -> [w329]
          shift-right: [w326] -> w322
          shift-left: errorcluster {"status"=FALSE, "code"=0, "source"=""} ("error out") -> [w327]
          tunnel: w319 -> [w328] mode=indexing
          tunnel: w318 -> [w331]
          n159 = Index Array(array=w331, index=w328) -> (element=w330:T2)
          n160 = Unbundle By Name(w330) -> ("Offset"=w325:i32)
          n161 = call "HH_SetInputChannelOffset.vi"("error in (no error)"=w327, "Offset"=w325, "channel"=w328, "devidx"=w329) -> ("error out"=w326:errorcluster)  [unwired: 6 in, 1 out]
        }
      }
      frame "SetInpChanTrg" {
        n162 = Unbundle By Name(w338) -> ("DevIdx"=w337:i32, "Channels"=w332:T2[], "CurrentChannels"=w333:i32[])
        n163 = for {
          tunnel: w337 -> [w341]
          shift-right: [w343] -> w336
          shift-left: errorcluster {"status"=FALSE, "code"=0, "source"=""} ("error out") -> [w344]
          tunnel: w333 -> [w342] mode=indexing
          tunnel: w332 -> [w346]
          n164 = Index Array(array=w346, index=w342) -> (element=w345:T2)
          n165 = Unbundle By Name(w345) -> ("CFDLevel"=w340:i32, "ZeroX"=w339:i32)
          n166 = call "HH_SetInputCFD.vi"("CFD Channel"=w342, "error in (no error)"=w344, "CFD ZeroCross"=w339, "CFD Level"=w340, "devidx"=w341) -> ("error out"=w343:errorcluster)  [unwired: 5 in, 1 out]
        }
      }
      frame "SetSyncDivider" {
        n167 = Unbundle By Name(w354) -> ("DevIdx"=w353:i32, "SyncDivider"=w349:i32)
        n168 = Power Of 2(x=w349) -> (2^x=w348:dbl)
        n169 = To Long Integer(number=w348) -> (32bit integer=w347:i32)
        n170 = call "HH_SetSyncDiv.vi"("SyncDivider"=w347, "devidx"=w353) -> ("error out"=w351:errorcluster)  [unwired: 8 in, 1 out]
        n171 = flat-sequence {
          tunnel: w351 -> [w355]
          tunnel: [w355] -> w350
          frame #0 {
            n172 = Wait (ms)(milliseconds to wait=u32 100) -> ()  [unwired: 1 out]
          }
        }
      }
      frame "SetSyncTrg" {
        n173 = Unbundle By Name(w362) -> ("DevIdx"=w359:i32, "SyncLevel"=w357:i32, "SyncZeroX"=w358:i32)
        n174 = call "HH_SetSyncCFD.vi"("CFD ZeroCross"=w358, "CFD Level"=w357, "devidx"=w359) -> ("error out"=w360:errorcluster)  [unwired: 7 in, 1 out]
      }
      frame "SetSyncOffset" {
        n175 = Unbundle By Name(w367) -> ("DevIdx"=w365:i32, "SyncOffset"=w364:i32)
        n176 = call "HH_SetSyncChannelOffset.vi"("Offset"=w364, "devidx"=w365) -> ("error out"=w366:errorcluster)  [unwired: 8 in, 1 out]
      }
      frame "SetBinning" {
        # "When binning is changed the new resolution is querried"
        n177 = Unbundle By Name(w374) -> ("DevIdx"=w372:i32, "Binning"=w371:i32)
        n178 = call "HH_SetBinning.vi"("Binning"=w371, "devidx"=w372) -> ("error out"=w373:errorcluster)  [unwired: 8 in, 1 out]
        n179 = Build Array (concatenate)(HH_UIThread_Cmds."GetResolution", w369) -> (w370:T10[])
      }
      frame "SetHistoOffset" {
        n180 = Unbundle By Name(w379) -> ("DevIdx"=w376:i32, "HistoOffset"=w375:i32)
        n181 = call "HH_SetOffset.vi"("Offset"=w375, "devidx"=w376) -> ("error out"=w377:errorcluster)  [unwired: 8 in, 1 out]
      }
      frame "SetStopOvl" {
        n182 = Unbundle By Name(w386) -> ("DevIdx"=w383:i32, "StopOvl."=w382:bool, "OvlLevel"=w381:u32)
        n183 = To Unsigned Long Integer(number=w381) -> (unsigned 32bit integer=w380:u32)
        n184 = call "HH_SetStopOverflow.vi"("stopcount"=w380, "StopOnOverflow"=w382, "devidx"=w383) -> ("error out"=w384:errorcluster)  [unwired: 7 in, 1 out]
      }
      frame "SetBitShift" {
        n185 = Unbundle By Name(w390) -> ("BitShift"=w388:i32, "SyncRate"=w389:i32)
        n186 = Negate(x=w388) -> (-x=w398:i32)
        n187 = Bundle By Name(cluster=T7 {"Cmd"=enum."Proc", "nActual"=0, "Buffer"=[], "TickCount"=0, "Param"=0} ("MH_DataProcThread_QData"), "Param"=w398, "Cmd"=HH_DataProcThread_QCmds."SetShift") -> (w404:T7)
        n188 = To Double Precision Float(number=w388) -> (double precision float=w403:dbl)
        n189 = To Double Precision Float(number=w389) -> (double precision float=w402:dbl)
        n190 = Power Of 2(x=w403) -> (2^x=w401:dbl)
        n191 = Enqueue Element(queue=w391, element=w404) -> ()  [unwired: 2 in, 3 out]
        n192 = Multiply(x=w401, y=1000.0) -> (x*y=w400:dbl)
        n193 = Divide(x=w400, y=w402) -> (x/y=w387:dbl)
        "DeltaT" <- w387
        n194 = Bundle By Name(cluster=T5 {"Histos"=[], "Cmd"=enum."_none_", "TimeTrace"=[], "Bin"=0, "Total bin"=0, "Status"="", "Resol"=0.0, "DeltaT"=0.0, "nChannels"=0} ("MH_GUIThread_QData"), "DeltaT"=w387, "Cmd"=HH_VisThread_QCmds."DeltaT") -> (w399:T5)
        n195 = Enqueue Element(queue=w392, element=w399) -> ()  [unwired: 2 in, 3 out]
      }
      frame "SetHistoAcqTime" {
        # "The time interval for accumulating a histogram from the photon stream is set on the front panel by the control labeled 'Int.Time  [s]' and saved to the UIThread Data cluster in the variable 'HistoAcqTime' (refer to case 'Idle' -> EventCase \"HistoAcqTime\": Value Change). Knowing the  SyncRate, from 'HistoAcqTime' the number of Sync-Pulses that would occur during that time intervall are calculated here and are send to 'HH_DataProcThread' by putting this number to 'Param' together with the command 'SetHistAcqTime' in the DataProcQ."
        n196 = Unbundle By Name(w407) -> ("SyncRate"=w413:i32, "HistoAcqTime"=w406:dbl)
        n197 = To Double Precision Float(number=w413) -> (double precision float=w416:dbl)
        n198 = Multiply(x=w416, y=w406) -> (x*y=w415:dbl)
        n199 = Round To Nearest(number=w415) -> (nearest integer value=w414:dbl)
        n200 = To Long Integer(number=w414) -> (32bit integer=w412:i32)
        n201 = Bundle By Name(cluster=T7 {"Cmd"=enum."Proc", "nActual"=0, "Buffer"=[], "TickCount"=0, "Param"=0} ("MH_DataProcThread_QData"), "Param"=w412, "Cmd"=HH_DataProcThread_QCmds."SetHistAcqTime") -> (w411:T7)
        n202 = Enqueue Element(queue=w408, element=w411) -> ()  [unwired: 2 in, 3 out]
      }
      frame "GetRates" {
        n203 = Unbundle By Name(w425) -> ("Init Info.nchannels"=w434:i32, "Channels"=w430:T2[], "DevIdx"=w421:i32, "StartMeas"=w428:bool, "SyncRateStart"=w419:i32)  [unwired: 1 out]
        n204 = call "HH_GetSyncRate.vi"("devidx"=w421) -> ("error out"=w423:errorcluster, "syncrate"=w420:i32)  [unwired: 8 in, 1 out]
        n205 = case shown="True" w428 {
          tunnel: w423 -> [w439 w442]
          tunnel: [w439 w444] -> w422
          tunnel: w420 -> [w438 _]
          tunnel: [w438 w449] -> w418
          tunnel: w419 -> [_ w440]
          tunnel: w427 -> [w437 w448]
          tunnel: [w437 w447] -> w426
          tunnel: w425 -> [w436 w446]
          tunnel: [w436 w445] -> w424
          tunnel: w421 -> [_ w441]
          frame False {
          }
          frame True {
            n206 = call "HH_GetSyncPeriod.vi"("error in (no error)"=w442, "devidx"=w441) -> ("error out"=w444:errorcluster, "period"=w443:dbl)  [unwired: 7 in, 1 out]
            n207 = Reciprocal(x=w443) -> (1/x=w450:dbl)
            n208 = To Long Integer(number=w450) -> (32bit integer=w449:i32)
            n209 = case shown="Default" w440 {
              selector: w440 -> [w451 _ _]
              tunnel: w449 -> [w454 w474 _]
              tunnel: w448 -> [w452 w477 w481]
              tunnel: [w453 w477 w481] -> w447
              tunnel: w446 -> [w458 w476 w480]
              tunnel: [w458 w475 w479] -> w445
              frame Default {
                n210 = Subtract(x=w454, y=w451) -> (x-y=w457:i32)
                n211 = Absolute Value(x=w457) -> (abs(x)=w455:i32)
                n212 = Not Equal To 0?(x=w455) -> (x != 0?=w456:bool)
                n213 = case shown="True" w456 {
                  tunnel: w455 -> [_ w467]
                  tunnel: [w459 w462] -> w453
                  tunnel: w452 -> [w459 w461]
                  tunnel: w451 -> [_ w460]
                  frame False {
                  }
                  frame True {
                    n214 = To Double Precision Float(number=w467) -> (double precision float=w466:dbl)
                    n215 = To Double Precision Float(number=w460) -> (double precision float=w468:dbl)
                    n216 = Divide(x=w466, y=w468) -> (x/y=w465:dbl)
                    n217 = Greater Or Equal?(x=w465, y=0.01) -> (x >= y?=w463:bool)
                    n218 = case shown="False" w463 {
                      tunnel: [w469 w472] -> w462
                      tunnel: w461 -> [w469 w470]
                      frame False {
                      }
                      frame True {
                        w471 = T10[] [enum."StopMeas"] items=["Idle", "Init", "SetInpChanEnable", "SetInpChanOffset", "SetInpChanTrg", "SetSyncDivider", "SetSyncTrg", "SetSyncOffset", "SetBinning", "SetHistoOffset", "SetHistoLen", "SetStopOvl", "SetBitShift", "SetHistoAcqTime", "GetRates", "StartMeas", "StopMeas", "AbortMeas", "GetResolution", "GetHisto", "ReadFiFo", "WriteStatus", "Resize", "EnableControls", "DisableControls", "Error", "Exit"]
                        n219 = One Button Dialog(message="Warning: Sync Rate has changed!\nTime Trace resolution has been changed accordingly.\nMeasurement is aborted.\n") -> ()  [unwired: 1 in, 1 out]
                        n220 = Build Array (concatenate)(w470, w471) -> (w472:T10[])
                      }
                    }
                  }
                }
              }
              frame -1 {
                n221 = Bundle By Name(cluster=w476, "SyncRateStart"=w474) -> (w475:T8)
              }
              frame -2 {
                n222 = Bundle By Name(cluster=w480, "SyncRateStart"=-1) -> (w479:T8)
              }
            }
          }
        }
        n223 = for {
          N: w434 -> [_]
          tunnel: w421 -> [w487]
          tunnel: [w484] -> w432 mode=indexing
          shift-right: [w486] -> w435
          shift-left: w422 -> [w488]
          tunnel: w430 -> [w483] mode=indexing
          i -> [w485]
          n224 = Unbundle By Name(w483) -> ("Enable"=w482:bool)
          n225 = case shown="True" w482 {
            tunnel: w488 -> [w489 w494]
            tunnel: w487 -> [_ w493]
            tunnel: [w489 w492] -> w486
            tunnel: w485 -> [_ w491]
            tunnel: [_ w490] -> w484
            frame False {
            }
            frame True {
              n226 = call "HH_GetCountRate.vi"("error in (no error)"=w494, "Channel"=w491, "devidx"=w493) -> ("error out"=w492:errorcluster, "rate"=w490:i32)  [unwired: 6 in, 1 out]
            }
          }
        }
        "CountRates" <- w432
        n227 = Format Into String(format string="Sync Rate: %d cps\n", w418) -> (resulting string=→"SyncRate":string)  [unwired: 2 in, 1 out]
        n228 = Bundle By Name(cluster=w424, "SyncRate"=w418) -> (w429:T8)
      }
      frame "StartMeas" {
        # "Starts the actual measurement by calling the driver function 'HH_StartMeas' and passing the acquisition time to it. Also the 'HH_DataProcThread' is initialized for a new measurement by putting the command 'Init' to the DataProcQ. The command 'ReadFiFo' is inserted to the UIThreads CmdQ (the shift register)."
        n229 = Bundle By Name(cluster=T7 {"Cmd"=enum."Proc", "nActual"=0, "Buffer"=[], "TickCount"=0, "Param"=0} ("MH_DataProcThread_QData"), "Cmd"=HH_DataProcThread_QCmds."Init") -> (w499:T7)
        n230 = Unbundle By Name(w497) -> ("DevIdx"=w506:i32, "AcqTime"=w502:i32)
        n231 = Enqueue Element(queue=w501, element=w499) -> ()  [unwired: 2 in, 3 out]
        n232 = Bundle By Name(cluster=w497, "SyncRateStart"=-2) -> (w496:T8)
        n233 = call "HH_StartMeas.vi"("tacq"=w502, "devidx"=w506) -> ("error out"=w507:errorcluster)  [unwired: 8 in, 1 out]
        n234 = Build Array (concatenate)(w505, HH_UIThread_Cmds."ReadFiFo") -> (w504:T10[])
      }
      frame "StopMeas" {
        n235 = Unbundle By Name(w513) -> ("Run cont."=w508:bool, "DevIdx"=w514:i32)
        n236 = call "HH_StopMeas.vi"("devidx"=w514) -> ("error out"=w515:errorcluster)  [unwired: 9 in, 1 out]
        n237 = case shown="False" w508 {
          tunnel: w513 -> [w519 w521]
          tunnel: [w518 w521] -> w512
          tunnel: [w516 w520] -> w511
          frame False {
            w516 = T10[] [enum."ReadFiFo"] items=["Idle", "Init", "SetInpChanEnable", "SetInpChanOffset", "SetInpChanTrg", "SetSyncDivider", "SetSyncTrg", "SetSyncOffset", "SetBinning", "SetHistoOffset", "SetHistoLen", "SetStopOvl", "SetBitShift", "SetHistoAcqTime", "GetRates", "StartMeas", "StopMeas", "AbortMeas", "GetResolution", "GetHisto", "ReadFiFo", "WriteStatus", "Resize", "EnableControls", "DisableControls", "Error", "Exit"]
            w517 = FALSE ("StartMeas")
            n238 = Bundle By Name(cluster=w519, "StartMeas"=w517) -> (w518:T8)
            n239 = local write "Start"(w517) -> ()
          }
          frame True {
            w520 = T10[] [enum."ReadFiFo", enum."StartMeas"] items=["Idle", "Init", "SetInpChanEnable", "SetInpChanOffset", "SetInpChanTrg", "SetSyncDivider", "SetSyncTrg", "SetSyncOffset", "SetBinning", "SetHistoOffset", "SetHistoLen", "SetStopOvl", "SetBitShift", "SetHistoAcqTime", "GetRates", "StartMeas", "StopMeas", "AbortMeas", "GetResolution", "GetHisto", "ReadFiFo", "WriteStatus", "Resize", "EnableControls", "DisableControls", "Error", "Exit"]
          }
        }
        n240 = Build Array (concatenate)(w510, w511) -> (w509:T10[])
      }
      frame "AbortMeas" {
        w523 = FALSE ("StartMeas")
        n241 = Unbundle By Name(w525) -> ("DevIdx"=w526:i32)
        n242 = call "HH_StopMeas.vi"("devidx"=w526) -> ("error out"=w527:errorcluster)  [unwired: 9 in, 1 out]
        n243 = Bundle By Name(cluster=w525, "StartMeas"=w523) -> (w524:T8)
        n244 = local write "Start"(w523) -> ()
      }
      frame "GetResolution" {
        # "Resolution in ns"
        # "Gets resolution in ps"
        # "Resolution is saved in UIThread Data cluster in ns"
        n245 = Unbundle By Name(w536) -> ("DevIdx"=w538:i32)
        n246 = call "HH_GetResolution.vi"("devidx"=w538) -> ("error out"=w537:errorcluster, "resolution"=w534:dbl)  [unwired: 8 in, 1 out]
        n247 = Divide(x=w534, y=1000.0) -> (x/y=w530:dbl)
        n248 = Bundle By Name(cluster=w536, "Resolution"=w530) -> (w535:T8)
        n249 = Bundle By Name(cluster=T5 {"Histos"=[], "Cmd"=enum."_none_", "TimeTrace"=[], "Bin"=0, "Total bin"=0, "Status"="", "Resol"=0.0, "DeltaT"=0.0, "nChannels"=0} ("MH_GUIThread_QData"), "Resol"=w530, "Cmd"=HH_VisThread_QCmds."Resol") -> (w528:T5)
        n250 = Enqueue Element(queue=w532, element=w528) -> ()  [unwired: 2 in, 3 out]
      }
      frame "ReadFiFo" {
        w548 = 2  # FLAG_FIFOFULL
        # "Reads photon records from HW and transferes them to DataProcThread via Queue."
        n251 = Unbundle By Name(w550) -> ("DevIdx"=w544:i32)
        n252 = call "HH_GetFlags.vi"("devidx"=w544) -> ("error out"=w546:errorcluster, "flags"=w547:i32)  [unwired: 8 in, 1 out]
        n253 = And(x=w547, y=w548) -> (x .and. y?=w549:i32)
        n254 = Not Equal To 0?(x=w549) -> (x != 0?=w543:bool)
        "OverRun" <- w543
        n255 = case shown="False" w543 {
          tunnel: w546 -> [w560 w563]
          tunnel: [w559 w563] -> w545
          tunnel: w544 -> [w552 _]
          tunnel: w542 -> [w558 _]
          tunnel: w541 -> [w557 _]
          tunnel: [w557 w561] -> w540
          frame False {
            n256 = call "HH_ReadFiFo.vi"("error in (no error)"=w560, "devidx"=w552) -> ("error out"=w559:errorcluster, "nactual"=w551:i32, "buffer"=w555:u32[])  [unwired: 6 in, 1 out]
            n257 = Bundle By Name(cluster=T7 {"Cmd"=enum."Proc", "nActual"=0, "Buffer"=[], "TickCount"=0, "Param"=0} ("MH_DataProcThread_QData"), "Buffer"=w555, "nActual"=w551, "Cmd"=HH_DataProcThread_QCmds."Proc") -> (w553:T7)
            n258 = Enqueue Element(queue=w558, element=w553) -> ()  [unwired: 2 in, 3 out]
          }
          frame True {
            n259 = Build Array(HH_UIThread_Cmds."AbortMeas") -> (w561:T10[])
          }
        }
      }
      frame "WriteStatus" {
        n260 = Unbundle By Name(w565) -> ("Status"=→"Status":string)
      }
      frame "Resize" {
        n261 = property on="Pane 3" class="Pane"() -> ("Width"=w572:u32)  [unwired: 2 in, 2 out]
        n262 = Subtract(x=w572, y=i16 100 ("b")) -> (x-y=w578:u32)
        n263 = Unbundle By Name(w567) -> ("Init Info.nchannels"=w575:i32)
        n264 = Quotient & Remainder(x=w578, y=i16 99 ("m")) -> (floor(x/y)=w577:u32)  [unwired: 1 out]
        n265 = In Range and Coerce(upper limit=w575, x=w577, lower limit=4) -> (coerced(x)=w576:u32)  [unwired: 1 out]
        n266 = Equal?(x=w575, y=w576) -> (x = y?=w574:bool)
        n267 = Not(x=w574) -> (.not. x?=w573:bool)
        n268 = property on="Channels" class="Arr (strict)"("HorizScroll"=w573, "Number of Columns"=w576, "Index Values"=u32[] [0]) -> ()  [unwired: 2 in, 2 out]
      }
      frame "EnableControls" {
        n269 = property class="VI"() -> ("Panel"=w583:refnum<vi>)  [unwired: 2 in, 2 out]
        n270 = property class="Pnl"(reference=w583) -> ("Controls[]"=w582:refnum<vi>[])  [unwired: 1 in, 2 out]
        n271 = property class="Pnl"(reference=w583) -> ("Decos[]"=w584:refnum<vi>[])  [unwired: 1 in, 2 out]
        n272 = for {
          tunnel: w584 -> [w588] mode=indexing
          tunnel: TRUE -> [w587]
          n273 = property class="Decor"(reference=w588, "Visible"=w587) -> ()  [unwired: 1 in, 2 out]
        }
        n274 = for {
          tunnel: w582 -> [w591] mode=indexing
          tunnel: T11."Enabled" ("Disabled") -> [w590]
          tunnel: [w589] -> _
          n275 = property class="Ctl"(reference=w591, "DisabledEnum"=w590) -> (error out=w589:errorcluster)  [unwired: 1 in, 1 out]
        }
      }
      frame "DisableControls" {
        n276 = property class="VI"() -> ("Panel"=w595:refnum<vi>)  [unwired: 2 in, 2 out]
        n277 = property class="Pnl"(reference=w595) -> ("Controls[]"=w594:refnum<vi>[])  [unwired: 1 in, 2 out]
        n278 = property class="Pnl"(reference=w595) -> ("Decos[]"=w596:refnum<vi>[])  [unwired: 1 in, 2 out]
        n279 = for {
          tunnel: w596 -> [w600] mode=indexing
          tunnel: FALSE -> [w599]
          n280 = property class="Decor"(reference=w600, "Visible"=w599) -> ()  [unwired: 1 in, 2 out]
        }
        n281 = for {
          tunnel: w594 -> [w603] mode=indexing
          tunnel: T11."Disabled and Grayed Out" ("Disabled") -> [w602]
          tunnel: [w601] -> _
          n282 = property class="Ctl"(reference=w603, "DisabledEnum"=w602) -> (error out=w601:errorcluster)  [unwired: 1 in, 1 out]
        }
      }
      frame "Error" {
        w604 = T10[] [enum."Exit"] items=["Idle", "Init", "SetInpChanEnable", "SetInpChanOffset", "SetInpChanTrg", "SetSyncDivider", "SetSyncTrg", "SetSyncOffset", "SetBinning", "SetHistoOffset", "SetHistoLen", "SetStopOvl", "SetBitShift", "SetHistoAcqTime", "GetRates", "StartMeas", "StopMeas", "AbortMeas", "GetResolution", "GetHisto", "ReadFiFo", "WriteStatus", "Resize", "EnableControls", "DisableControls", "Error", "Exit"]
        w607 = T14 1 items=["no dialog", "OK message", "continue or stop message", "OK message + warnings", "continue/stop + warnings"] ("type of dialog (OK msg:1)")
        # "Error case: If an error occures the user is informed and the programm terminates. Add your own code to handle error events (e.g. exception lists, etc.)"
        n283 = call <vilib>:"Simple Error Handler.vi"("type of dialog (OK msg:1)"=w607, "error in (no error)"=w606) -> ()  [unwired: 3 in, 5 out]
      }
      frame "Exit" {
        n284 = Release Queue(queue=w609) -> ()  [unwired: 2 in, 3 out]
        n285 = Release Queue(queue=w608) -> ()  [unwired: 2 in, 3 out]
        n286 = Unbundle By Name(w613) -> ("DevIdx"=w612:i32)
        n287 = call "HH_CloseDevice.vi"("devidx"=w612) -> ("error out"=w611:errorcluster)  [unwired: 9 in, 1 out]
      }
    }
    n288 = call "HH_EnQError.vi"("error in (no error)"=w24, "Cmds_in"=w22) -> ("error out"=w23:errorcluster, "Cmds_out"=w21:T10[])  [unwired: 8 in]
  }
  n289 = call "HH_DataProcThread.vi"("HH_VisThread_QRef"=w7, "HH_DataProcThread_QRef"=w1) -> ()  [unwired: 10 in]
  n290 = while {
    tunnel: w7 -> [w622]
    shift-right: [w618] -> _
    shift-left: T4 {"Resol"=0.0, "DeltaT"=0.0, "NumChannels"=0} -> [w619]
    tunnel: w1 -> [w617]
    stop <- w615 stop-if-true
    # "VisualizationThread"
    n291 = Dequeue Element(queue=w622, timeout in ms (-1)=100) -> (element=w620:T5, error out=w615:errorcluster)  [unwired: 1 in, 2 out]
    n292 = Unbundle By Name(w620) -> ("Cmd"=w621:T6)
    n293 = case shown="\"DeltaT\"" w621 {
      tunnel: w620 -> [_ w635 w637 w649 w657 w661 w665]
      tunnel: w619 -> [w625 w633 w639 w641 w656 w660 w664]
      tunnel: [w625 w633 w638 w641 w656 w659 w663] -> w618
      tunnel: w617 -> [w624 _ _ _ w653 _ _]
      tunnel: w615 -> [w623 _ _ _ _ _ _]
      frame "_none_", Default {
        n294 = case shown="No Error" w623 {
          tunnel: w624 -> [w629 _]
          frame No Error {
            n295 = Get Queue Status(queue=w629) -> (# elements in queue=w627:i32)  [unwired: 2 in, 7 out]
            n296 = Format Into String(format string="Elements in Q: %d", w627) -> (resulting string=w626:string)  [unwired: 2 in, 1 out]
            n297 = local write "Status"(w626) -> ()
          }
          frame Error {
          }
        }
      }
      frame "Histo" {
        n298 = Unbundle By Name(w635) -> ("Histos"=w630:u32[][])
        n299 = Unbundle By Name(w633) -> ("Resol"=w632:dbl)
        n300 = Bundle(0.0, "Resol"=w632, "Histos"=w630) -> (→"HistoGraph":cluster{dbl, "Resol":dbl, "Histos":u32[][]})  [unwired: 1 in]
      }
      frame "nChannels" {
        n301 = Unbundle By Name(w637) -> ("nChannels"=w636:i32)
        n302 = Bundle By Name(cluster=w639, "NumChannels"=w636) -> (w638:T4)
      }
      frame "TTrace" {
        n303 = Unbundle By Name(w649) -> ("Total bin"=w648:u64, "Bin"=w647:i32, "TimeTrace"=w646:u32[][])
        n304 = Unbundle By Name(w641) -> ("DeltaT"=w640:dbl)
        n305 = call "HH_TTraceToGraph.vi"("DeltaT"=w640, "TimeTrace"=w646, "Bin"=w647, "Total bin"=w648) -> ("TimeTrace_out"=w643:u32[][], "dt"=w644:dbl, "T0"=w645:dbl)  [unwired: 5 in]
        n306 = Bundle("T0"=w645, "dt"=w644, "TimeTrace_out"=w643) -> (→"TTraceGraph":T15)  [unwired: 1 in]
      }
      frame "Status" {
        n307 = Unbundle By Name(w657) -> ("Status"=w654:string)
        n308 = Get Queue Status(queue=w653) -> (# elements in queue=w652:i32)  [unwired: 2 in, 7 out]
        n309 = Format Into String(format string="\t\tElements in Q: %d", w652) -> (resulting string=w650:string)  [unwired: 2 in, 1 out]
        n310 = Concatenate Strings(w654, w650) -> (w655:string)
        n311 = local write "Status"(w655) -> ()
      }
      frame "DeltaT" {
        n312 = Unbundle By Name(w661) -> ("DeltaT"=w658:dbl)
        n313 = Bundle By Name(cluster=w660, "DeltaT"=w658) -> (w659:T4)
      }
      frame "Resol" {
        n314 = Unbundle By Name(w665) -> ("Resol"=w662:dbl)
        n315 = Bundle By Name(cluster=w664, "Resol"=w662) -> (w663:T4)
      }
    }
  }
